vi "Rec Fetch Next Recordset (R).vi"(4 "error in (no error)":errorcluster, 7 "recordset reference":T1) -> (0 "error out":errorcluster, 3 "recordset reference out":T1)   [LabVIEW 2020, in "NI_Database_API.lvlib"]
doc: "Retrieves the next recordset in a multi-recordset query identified by <B>recordset reference</B>. When the current recordset is no longer available, the <B>recordset reference</B> is redirected to the new recordset. Wire data to the reference input to determine the polymorphic instance to use or manually select the instance."
uses:
  <vilib>/addons/database/NI_Database_API.lvlib
  <vilib>/addons/database/Recordset.llb/Rec ObjectReference.ctl
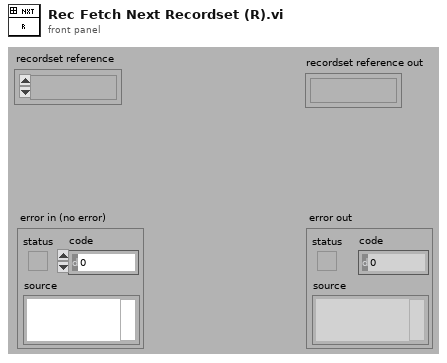
[diagram p1: front panel]
types:
  T1 = typedef "NI_Database_API.lvlib/Rec ObjectReference.ctl" = refnum<k1>
  T2 = typedef "NI_Database_API.lvlib/Rec DataMembers.ctl" = cluster{"ADODB._Recordset":refnum<k7>, "Connection":T3}
  T3 = typedef "NI_Database_API.lvlib/Conn ObjectReference.ctl" = refnum<k1>
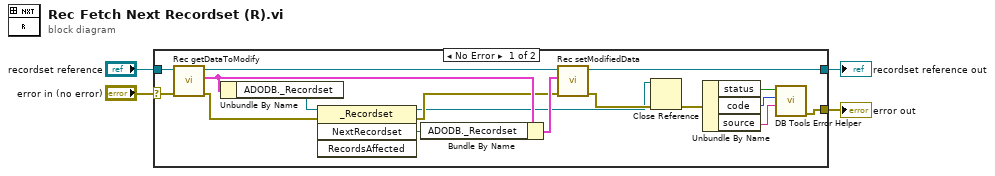
[diagram p0: block diagram]
diagram:
  n1 = case shown="No Error" "error in (no error)" {
    selector: "error in (no error)" -> [w8 w23]
    tunnel: "recordset reference" -> [w20 w22]
    tunnel: [w13 w22] -> w3
    tunnel: [w9 w23] -> w2
    frame No Error {
      n2 = call <vilib>:"Rec getDataToModify.vi"("error in (no error)"=w8, "recordset reference"=w20) -> ("error out"=w17:errorcluster, "data"=w21:T2, "recordset reference out"=w14:T1)  [unwired: 3 out]
      n3 = Unbundle By Name(w21) -> ("ADODB._Recordset"=w18:refnum<k7>)
      n4 = invoke class="_Recordset" method="NextRecordset"(reference=w18, error in=w17) -> (reference out=w5:refnum<k7>, error out=w15:errorcluster, "NextRecordset"=w16:refnum<k7>)  [unwired: 2 in, 1 out]
      n5 = Bundle By Name(cluster=w21, "ADODB._Recordset"=w16) -> (w19:T2)
      n6 = call <vilib>:"Rec setModifiedData.vi"("error in (no error)"=w15, "data"=w19, "recordset reference"=w14) -> ("error out"=w6:errorcluster, "recordset reference out"=w13:T1)  [unwired: 3 out]
      n7 = Close Reference(reference=w5, error in (no error)=w6) -> (error out=w7:errorcluster)
      n8 = Unbundle By Name(w7) -> ("status"=w11:bool, "code"=w10:i32, "source"=w12:string)
      n9 = call <vilib>:"DB Tools Error Helper.vi"("source"=w12, "code"=w10, "status"=w11) -> ("error out"=w9:errorcluster)  [unwired: 1 in, 7 out]
    }
    frame Error {
    }
  }
  "recordset reference out" <- w3
  "error out" <- w2
